vi "Send Create SV.vi"(6 "Mode (commit)":u16(ring) items=["commit", "buffer"], 7 "Message Priority (Normal)":T1=enum."Normal", 8 "error in (no error)":errorcluster, 9 "shared variable name":string, 10 "process name":string, 11 "Message Enqueuer":refnum<class "Message Enqueuer.lvclass">) -> (0 "error out":errorcluster, 3 "Message Enqueuer out":refnum<class "Message Enqueuer.lvclass">)   [LabVIEW 2015, in "CS++DSCManager.lvlib" / "Create SV Msg.lvclass"]
doc: "Sends the <B>CS++DSCManager.lvlib:Create SV Msg.lvclass</B> message.\n\n<B>CS++DSCManager.lvlib:CS++DSCManager.lvclass:Create SV.vi</B> Description:\n\nCreates a shared variable of the given name and type in the specified process. The shared variable that you want to create replaces an existing shared variable if the two shared variables have the same name."
uses:
  Create SV Msg.lvclass
  <vilib>/ActorFramework/Message Enqueuer/Message Enqueuer.lvclass
  <vilib>/ActorFramework/Message Enqueuer/Message Priority.ctl
  Create SV Msg.lvclass/Create SV Msg.ctl
  <vilib>/ActorFramework/Message Enqueuer/Message Enqueuer.lvclass/Message Enqueuer.ctl
  <vilib>/ActorFramework/Message Priority Queue/Priority Enqueue.vi
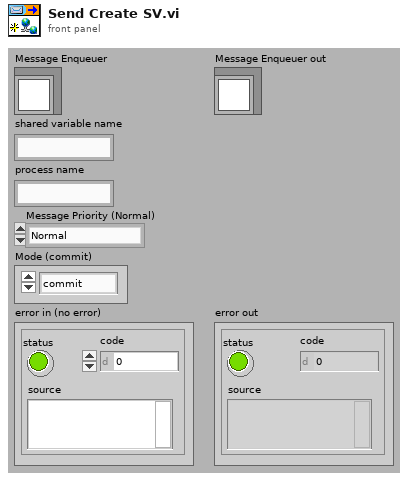
[diagram p1: front panel]
types:
  T1 = typedef "Actor Framework.lvlib/Message Enqueuer.lvclass/Message Priority.ctl" = enum16{"Low", "Normal", "High"}
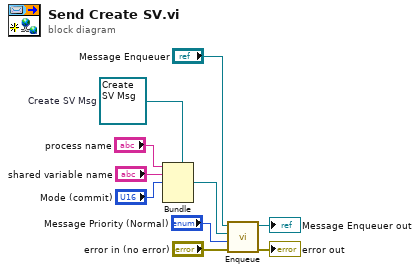
[diagram p0: block diagram]
diagram:
  w4 = refnum<class "Create SV Msg.lvclass"> refnum  # Create SV Msg
  n1 = Bundle(cluster=w4, "process name", "shared variable name", "Mode (commit)") -> (w7:refnum<class "Create SV Msg.lvclass">)  [unwired: 2 in]
  n2 = call <vilib>:"Enqueue.vi"("error in (no error)"="error in (no error)", "Message Priority (Normal)"="Message Priority (Normal)", "Message"=w7, "Message Enqueuer in"="Message Enqueuer") -> ("error out"=→"error out":errorcluster, "Message Enqueuer out"=→"Message Enqueuer out":refnum<class "Message Enqueuer.lvclass">)  [unwired: 6 in]
